vi "read TBM configuration.vi"(8 "error in":errorcluster, 11 "Systems in":refnum<class "Systems.lvclass">) -> (0 "error out":errorcluster, 2 "configuration":refnum<class "TBM configuration.lvclass">, 3 "Systems out":refnum<class "Systems.lvclass">)   [LabVIEW 2013, in "PL Framework Configuration Tool.lvlib" / "Systems.lvclass"]
uses:
  Systems.lvclass
  <vilib>/NI/Tag Bus Module Framework/root configuration/TBM configuration.lvclass
  Systems.lvclass/Systems.ctl
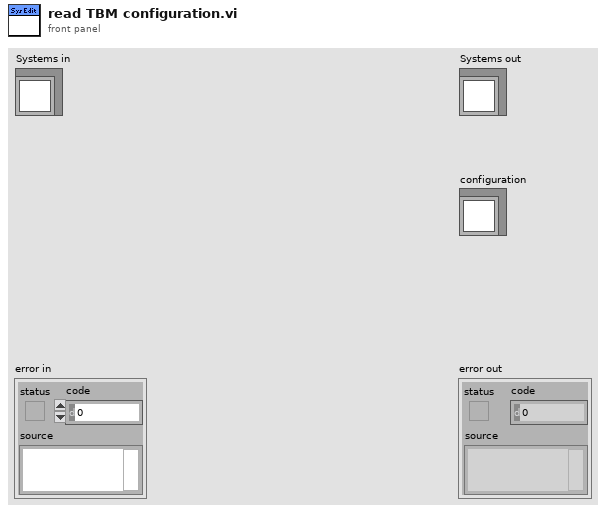
[diagram p1: front panel]
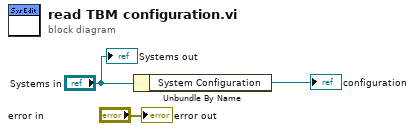
[diagram p0: block diagram]
diagram:
  n1 = Unbundle By Name("Systems in") -> ("System Configuration"=→"configuration":refnum<class "PL_System Configuration.lvclass">)
  "error out" <- "error in"
  "Systems out" <- "Systems in"
